vi "IOCtrl_setAllOutputs.vi"(8 "error in (no error)":errorcluster) -> (0 "error out":errorcluster)   [LabVIEW 2015, in "ESLSCDLL.lvlib"]
uses:
  ESLSCDLL.lvlib
  Globals.vi
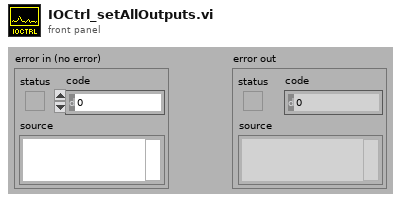
[diagram p1: front panel]
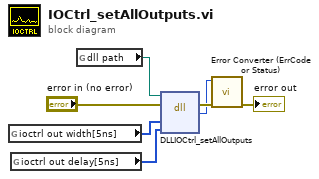
[diagram p0: block diagram]
diagram:
  n1 = global read "Globals.vi" "ioctrl out width[5ns]"() -> (w3:u32[])
  n2 = global read "Globals.vi" "ioctrl out delay[5ns]"() -> (w2:u32[])
  n3 = global read "Globals.vi" "dll path"() -> (w1:path)
  n4 = dll-call lib="C:/ENTW/PCIE/LV64/board.vis/ESLSCDLL.dll" fn="DLLIOCtrl_setAllOutputs" ("lwlscdll.dll:DLLSetTemp")(path in=w1, error in="error in (no error)", "width_in_5ns"=w3, "delay_in_5ns"=w2) -> (error out=w6:errorcluster, "es_status_codes"=w4:i32)  [unwired: 3 in, 1 out]
  n5 = call "Error Converter (ErrCode or Status).vi"("error in (no error)"=w6, "error code"=w4) -> ("error out"=→"error out":errorcluster)  [unwired: 9 in]
